vi "sslSimulationProtocolDecodeSimulatorError.vi"(8 "error in":errorcluster, 10 "Key":i32=1, 11 "robotControlResponseArray":u8[](array[numeric])) -> (0 "error out":errorcluster, 3 "array w/ subset deleted":u8[](array[numeric]))   [LabVIEW 2020, in "Communication.lvclass"]
uses:
  Communication.lvclass
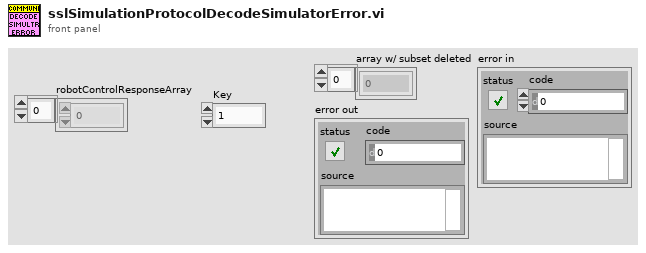
[diagram p1: front panel]
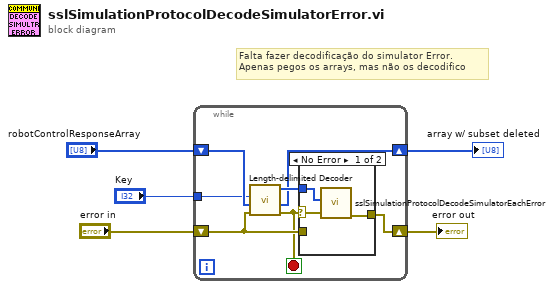
[diagram p0: block diagram]
diagram:
  # "Falta fazer decodificação do simulator Error.\nApenas pegos os arrays, mas não os decodifico"
  n1 = while {
    shift-right: [w10] -> w3
    shift-left: "robotControlResponseArray" -> [w7]
    shift-right: [w12] -> w1
    shift-left: "error in" -> [w9]
    tunnel: "Key" -> [w6]
    stop <- w8 stop-if-true
    n2 = call "Length-delimited Decoder.vi"("error in (no error)"=w9, "Array"=w7, "Key"=w6) -> ("error out"=w8:errorcluster, "array w/ subset deleted"=w10:u8[], "Length-delimited"=w11:u8[])  [unwired: 5 in, 1 out]
    n3 = case shown="No Error" w8 {
      selector: w8 -> [w15 _]
      tunnel: [w14 w16] -> w12
      tunnel: w11 -> [w13 _]
      tunnel: w9 -> [_ w16]
      frame No Error {
        n4 = call "sslSimulationProtocolDecodeSimulatorEachError.vi"("error in (no error)"=w15, "simulatorErrorArray"=w13) -> ("error out"=w14:errorcluster)  [unwired: 8 in, 1 out]
      }
      frame Error {
      }
    }
  }
  "array w/ subset deleted" <- w3
  "error out" <- w1
